vi "resize.vi"(6 "fill with (0x0)":u8 format="%.0x", 8 "error in (no error)":errorcluster, 9 "new_size (from offset)":i32, 10 "offset (-1: current position)":i32=-1, 11 "Bytes in":refnum<class "Bytes.lvclass">) -> (0 "error out":errorcluster, 2 "total_size":i32, 3 "Bytes out":refnum<class "Bytes.lvclass">)   [LabVIEW 2020, in "lvdata.lvlib" / "Bytes.lvclass"]
uses:
  Bytes.lvclass
  Bytes.lvclass/Bytes.ctl
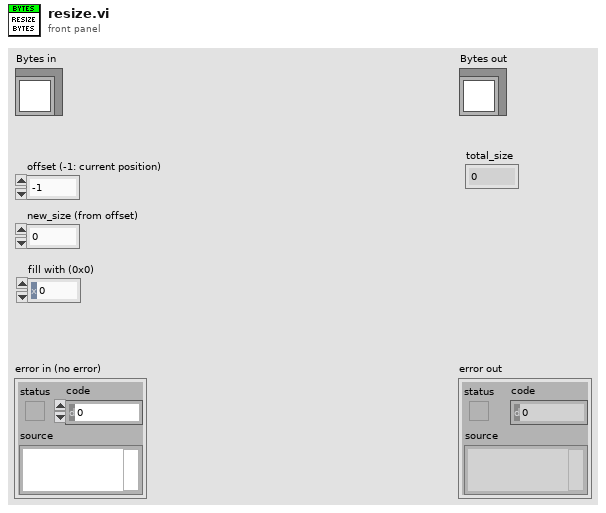
[diagram p1: front panel]
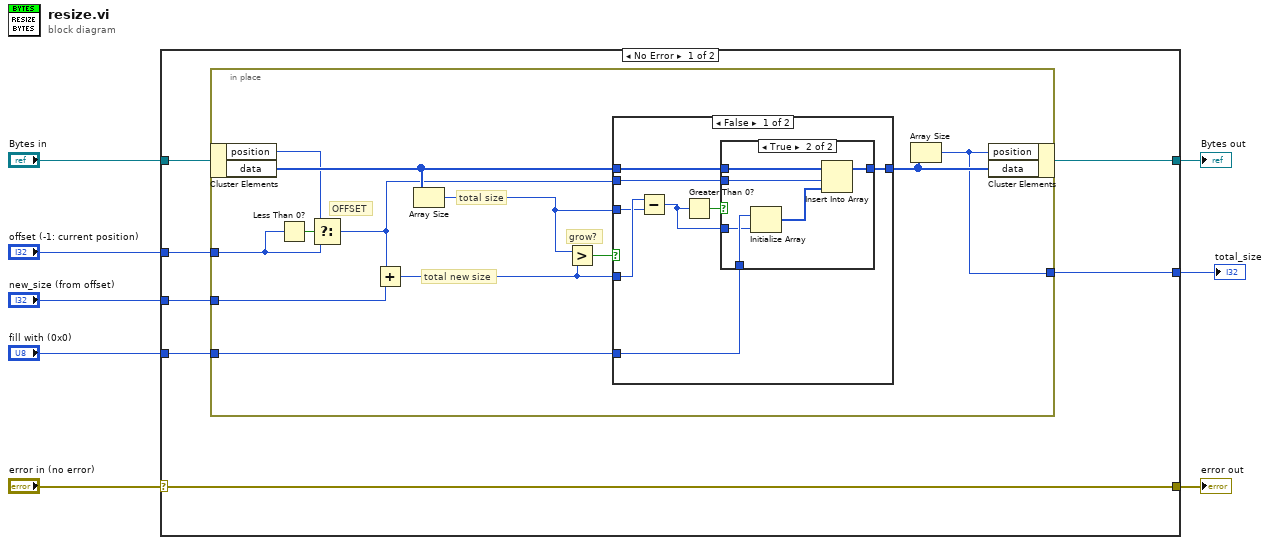
[diagram p0: block diagram]
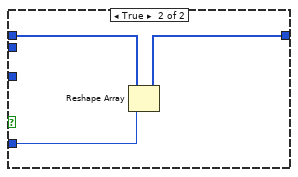
[diagram p3: hidden frame]
diagram:
  n1 = case shown="No Error" "error in (no error)" {
    selector: "error in (no error)" -> [w15 w47]
    tunnel: [w15 w47] -> w7
    tunnel: [w14 w46] -> w5
    tunnel: "Bytes in" -> [w11 w46]
    tunnel: "new_size (from offset)" -> [w13 _]
    tunnel: "fill with (0x0)" -> [w12 _]
    tunnel: "offset (-1: current position)" -> [w10 _]
    tunnel: [w9 _] -> w1
    frame No Error {
      n2 = in-place {
        in-place-border: w13 -> [w23]
        in-place-border: w12 -> [w25]
        in-place-border: w10 -> [w20]
        in-place-border: [w16] -> w9
        # "grow?"
        # "total size"
        # "total new size"
        # "OFFSET"
        n3 = in-place-cluster #1(w11) -> ("position"=w18:i32, "data"=w27:u8[])
        n4 = Less Than 0?(x=w20) -> (x < 0?=w21:bool)
        n5 = Select(t=w18, s=w21, f=w20) -> (s? t:f=w19:i32)
        n6 = Add(x=w19, y=w23) -> (x+y=w22:i32)
        n7 = Array Size(array=w27) -> (size(s)=w24:i32)
        n8 = Greater?(x=w24, y=w22) -> (0:w26:bool)
        n9 = case shown="False" w26 {
          tunnel: w27 -> [w33 w43]
          tunnel: [w32 w44] -> w17
          tunnel: w22 -> [w35 w45]
          tunnel: w25 -> [w30 _]
          tunnel: w19 -> [w31 _]
          tunnel: w24 -> [w34 _]
          frame False {
            n10 = Subtract(x=w35, y=w34) -> (x-y=w29:i32)
            n11 = Greater Than 0?(x=w29) -> (x > 0?=w28:bool)
            n12 = case shown="True" w28 {
              tunnel: w33 -> [w36 w42]
              tunnel: [w36 w41] -> w32
              tunnel: w31 -> [_ w40]
              tunnel: w30 -> [_ w39]
              tunnel: w29 -> [_ w38]
              frame False {
              }
              frame True {
                n13 = Initialize Array(w39, w38) -> (w37:u8[])
                n14 = Insert Into Array(array=w42, index=w40, new element=w37) -> (w41:u8[])
              }
            }
          }
          frame True {
            n15 = Reshape Array(w43, w45) -> (w44:u8[])
          }
        }
        n16 = Array Size(array=w17) -> (size(s)=w16:i32)
        n17 = in-place-cluster #1("position"=w16, "data"=w17) -> (w14:refnum<class "Bytes.lvclass">)
      }
    }
    frame Error {
    }
  }
  "error out" <- w7
  "Bytes out" <- w5
  "total_size" <- w1
